vi "Playback Controls.vi"() -> ()   [LabVIEW 2020]
uses:
  <vilib>/Rock Robotics/WPI/Dashboard/WPI_DashboardPlay Operation.ctl
  <vilib>/Rock Robotics/WPI/Dashboard/WPI_DashboardLogging Global.vi
  <vilib>/Utility/inputDevices.llb/mouseAcquire.vi
panel:
  in  "Operation":u16(ring) items=["", "Rename", "Delete", "Show Folder"]
  in  "Rename":string
  in  "Dragging?":bool
  in  "Scrollbar":dbl(slide) scale=0.0..12.36
  in  "Speed":u16(ring)=3 items=["1/10 x", "1/5 x", "1/2 x", "1 x", "2 x", "5 x", "10 x"]
  in  "Playback Button":bool
  in  "Pause Button":bool
  in  "File Selector":u16(ring) items=["Select a Log File", "2017_11_07 07-17-37 Tue -- 3.2 secs", "2017_11_07 08-09-29 Tue -- 8.7 secs", "2017_11_07 08-19-10 Tue -- 11.1 secs", "2017_11_07 08-21-00 Tue -- 12.4 secs", "Test -- 2.6 secs"]
  in  "Drag Button":bool
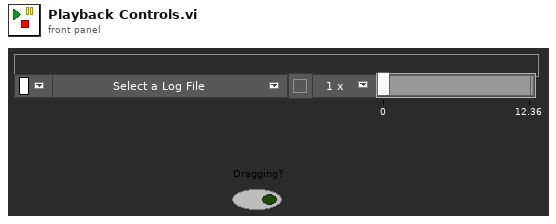
[diagram p1: front panel]
types:
  T1 = cluster{"Video 1":i32, "Video 2":i32, "Video 3":i32, "Video 4":i32}
  T2 = typedef "WPI_DashboardPlay Operation.ctl" = enum16{"Play", "Pause", "Finished"}
  T3 = typedef "LVRectTypeDef.ctl" = cluster{"Left":i16, "Top":i16, "Right":i16, "Bottom":i16}
  T4 = cluster{"Horizontal":i32, "Vertical":i32, "Scrolling":i32}
  T5 = cluster{"Horizontal":i32, "Vertical":i32, "Horizontal":i32, "Vertical":i32}
  T6 = cluster{"button 1":bool, "button 2":bool, "button 3":bool, "button 4":bool}
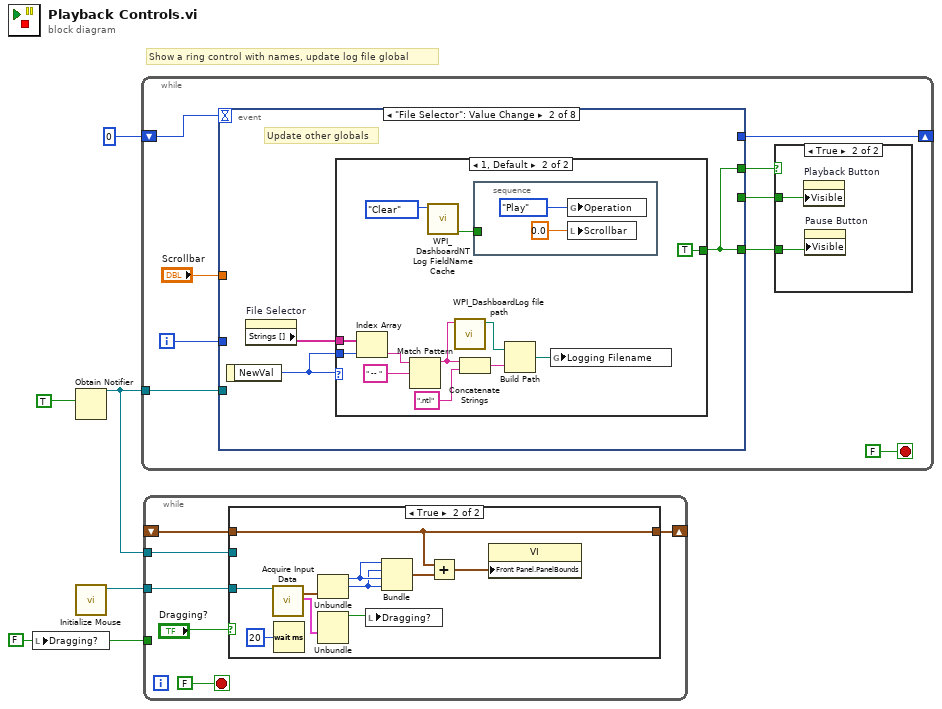
[diagram p0: block diagram]
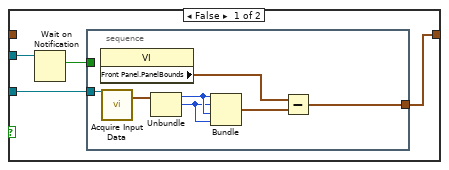
[diagram p2: hidden frame]
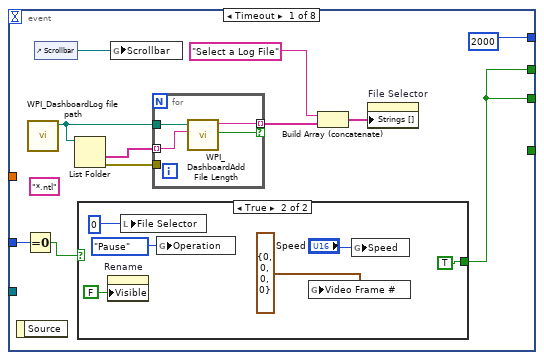
[diagram p4: hidden frame]
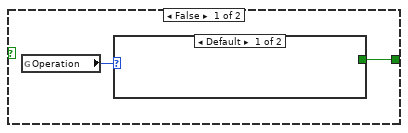
[diagram p5: hidden frame]
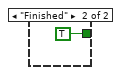
[diagram p6: hidden frame]
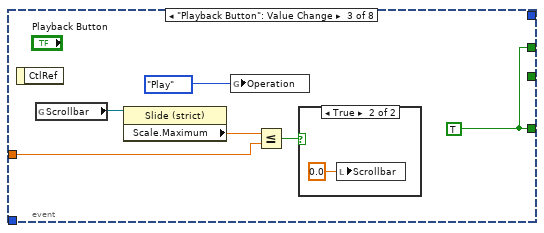
[diagram p8: hidden frame]
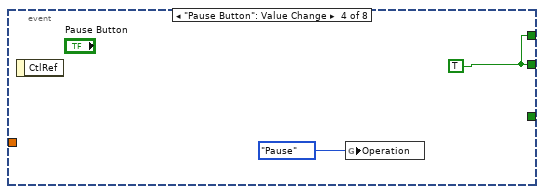
[diagram p10: hidden frame]
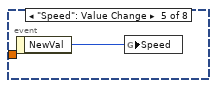
[diagram p11: hidden frame]
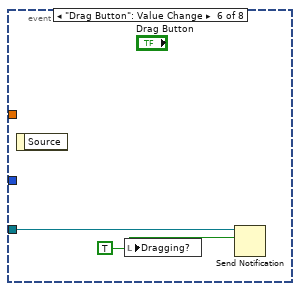
[diagram p12: hidden frame]
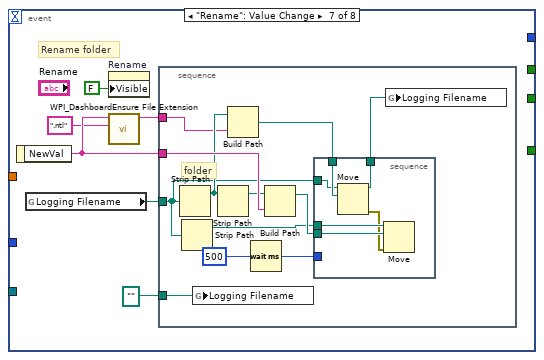
[diagram p13: hidden frame]
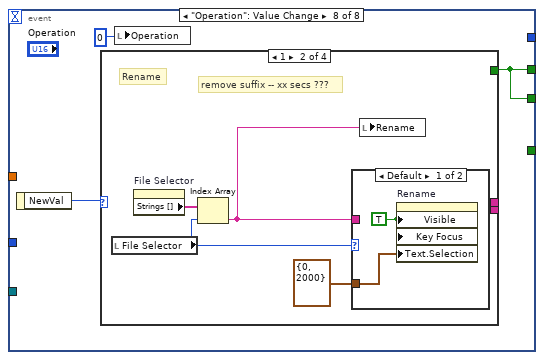
[diagram p14: hidden frame]
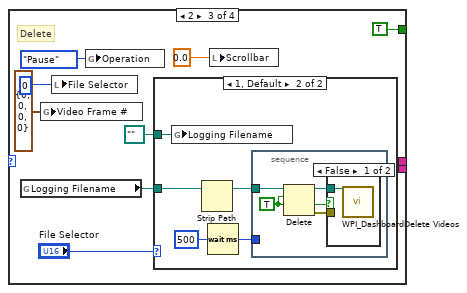
[diagram p17: hidden frame]
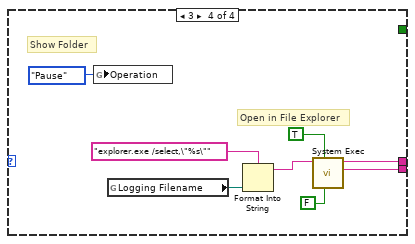
[diagram p20: hidden frame]
diagram:
  w2 = FALSE ("Dragging?")
  # "Show a ring control with names, update log file global"
  n1 = local write "Dragging?"(w2) -> ()
  n2 = Obtain Notifier(notification data type=TRUE ("Dragging?")) -> (notifier out=w3:refnum<notifier>)  [unwired: 3 in, 2 out]
  n3 = call <vilib>:"Initialize Mouse.vi"() -> ("device ID"=w4:refnum<k1>)  [unwired: 10 in, 1 out]
  n4 = while {
    shift-right: [w13] -> _
    shift-left: 0 -> [w12]
    tunnel: w3 -> [w6]
    i -> [w8]
    stop <- FALSE stop-if-true
    n5 = event shown="[1] \"File Selector\": Value Change" {
      selector: _ -> [_ _ _ _ _ _ _ _]
      dyn-events: _ -> [_ _ _ _ _ _ _ _]
      timeout: w12 -> [_ _ _ _ _ _ _ _]
      tunnel: [2000 _ _ _ _ _ _ _] -> w13
      tunnel: [_ w41 w63 _ _ _ _ _] -> w11
      tunnel: [w20 _ _ w66 _ _ _ w95] -> w10
      tunnel: [w20 w41 w63 w66 _ _ _ w95] -> w9
      tunnel: w8 -> [w22 _ _ _ _ _ _ _]
      tunnel: "Scrollbar" -> [_ _ w59 _ _ _ _ _]
      tunnel: w6 -> [_ _ _ _ _ w69 _ _]
      event Timeout {
        (unwired) "*.ntl" ("pattern")
        n6 = event-data() -> ()  [unwired: 1 in, 1 out]
        n7 = Equal To 0?(x=w22) -> (x = 0?=w21:bool)
        n8 = call <vilib>:"WPI_DashboardLog file path.vi"() -> ("appended path"=w19:path)  [unwired: 11 in]
        n9 = control-ref of="Scrollbar"() -> (w26:refnum<vi>)
        n10 = List Folder(path=w19) -> (folder names=w17:string[], error out=w18:errorcluster)  [unwired: 3 in, 2 out]
        n11 = case shown="True" w21 {
          tunnel: [w28 TRUE] -> w20
          frame False {
            n12 = global read "WPI_DashboardLogging Global.vi" "Operation"() -> (w29:T2)
            n13 = case shown="Default" w29 {
              tunnel: [_ TRUE] -> w28
              frame Default {
              }
              frame "Finished" {
              }
            }
          }
          frame True {
            n14 = property on="Rename" class="Str"("Visible"=FALSE) -> ()  [unwired: 2 in, 2 out]
            n15 = local write "File Selector"(0) -> ()
            n16 = global write "WPI_DashboardLogging Global.vi" "Operation"(WPI_DashboardPlay_Operation."Pause" ("Operation")) -> ()
            n17 = global write "WPI_DashboardLogging Global.vi" "Video Frame #"(T1 {"Video 1"=0, "Video 2"=0, "Video 3"=0, "Video 4"=0} ("Video Frame #")) -> ()
            n18 = global write "WPI_DashboardLogging Global.vi" "Speed"("Speed") -> ()
          }
        }
        n19 = global write "WPI_DashboardLogging Global.vi" "Scrollbar"(w26) -> ()
        n20 = for {
          tunnel: w17 -> [w38] mode=indexing
          tunnel: [w40] -> w25 mode=indexing if=w37
          tunnel: w19 -> [w39]
          tunnel: w18 -> [_]
          n21 = call <vilib>:"WPI_DashboardAdd File Length.vi"("String in"=w38, "appended path"=w39) -> ("Valid"=w37:bool, "String out"=w40:string)  [unwired: 8 in]
        }
        n22 = Build Array (concatenate)("Select a Log File" ("pattern"), w25) -> (w24:string[])
        n23 = property on="File Selector" class="Ring (strict)"("Strings []"=w24) -> ()  [unwired: 2 in, 2 out]
      }
      event "File Selector": Value Change {
        # "Update other globals"
        n24 = event-data() -> ("NewVal"=w42:u16)  [unwired: 1 in]
        n25 = property on="File Selector" class="Ring (strict)"() -> ("Strings []"=w43:string[])  [unwired: 2 in, 2 out]
        n26 = case shown="1, Default" w42 {
          tunnel: w43 -> [_ w55]
          tunnel: w42 -> [_ w54]
          tunnel: [_ TRUE ("Visible")] -> w41
          frame 0 {
          }
          frame 1, Default {
            n27 = Index Array(array=w55, index=w54) -> (element=w49:string)
            n28 = Match Pattern(string=w49, regular expression=" -- ") -> (before substring=w44:string)  [unwired: 1 in, 3 out]
            n29 = call <vilib>:"WPI_DashboardNT Log FieldName Cache.vi"("Operation"=enum16{"Lookup/Add", "Index", "Clear"}."Clear") -> ("New/Valid"=w46:bool)  [unwired: 8 in, 2 out]
            n30 = call <vilib>:"WPI_DashboardLog file path.vi"("Time Date String"=w44) -> ("appended path"=w53:path)  [unwired: 10 in]
            n31 = Concatenate Strings(w44, ".ntl") -> (w51:string)
            n32 = stacked-sequence {
              tunnel: w46 -> [_]
              frame #0 {
                n33 = global write "WPI_DashboardLogging Global.vi" "Operation"(WPI_DashboardPlay_Operation."Play" ("Operation")) -> ()
                n34 = local write "Scrollbar"(0.0 ("Position")) -> ()
              }
            }
            n35 = Build Path(base path=w53, name or relative path=w51) -> (appended path=w50:path)
            n36 = global write "WPI_DashboardLogging Global.vi" "Logging Filename"(w50) -> ()
          }
        }
      }
      event "Playback Button": Value Change {
        w63 = TRUE ("Visible")
        n37 = event-data() -> ()  [unwired: 1 in, 1 out]
        n38 = global read "WPI_DashboardLogging Global.vi" "Scrollbar"() -> (w61:refnum<vi>)
        n39 = property class="Slide (strict)"(reference=w61) -> ("Scale.Maximum"=w60:dbl)  [unwired: 1 in, 2 out]
        n40 = global write "WPI_DashboardLogging Global.vi" "Operation"(WPI_DashboardPlay_Operation."Play" ("Operation")) -> ()
        n41 = Less Or Equal?(x=w60, y=w59) -> (x <= y?=w58:bool)
        n42 = case shown="True" w58 {
          frame False {
          }
          frame True {
            n43 = local write "Scrollbar"(0.0 ("Scrollbar")) -> ()
          }
        }
      }
      event "Pause Button": Value Change {
        w66 = TRUE ("Visible")
        n44 = event-data() -> ()  [unwired: 1 in, 1 out]
        n45 = global write "WPI_DashboardLogging Global.vi" "Operation"(WPI_DashboardPlay_Operation."Pause" ("Operation")) -> ()
      }
      event "Speed": Value Change {
        n46 = event-data() -> ("NewVal"=w67:u16)  [unwired: 1 in]
        n47 = global write "WPI_DashboardLogging Global.vi" "Speed"(w67) -> ()
      }
      event "Drag Button": Value Change {
        w68 = TRUE ("Dragging?")
        n48 = event-data() -> ()  [unwired: 1 in, 1 out]
        n49 = local write "Dragging?"(w68) -> ()
        n50 = Send Notification(notification=w68, notifier=w69) -> ()  [unwired: 1 in, 2 out]
      }
      event "Rename": Value Change {
        # "Rename folder"
        n51 = event-data() -> ("NewVal"=w72:string)  [unwired: 1 in]
        n52 = global read "WPI_DashboardLogging Global.vi" "Logging Filename"() -> (w74:path)
        n53 = property on="Rename" class="Str"("Visible"=FALSE) -> ()  [unwired: 2 in, 2 out]
        n54 = call <vilib>:"WPI_DashboardEnsure File Extension.vi"("Extension"=".ntl", "Name"=w72) -> ("Name Out"=w70:string)  [unwired: 9 in]
        n55 = stacked-sequence {
          tunnel: w72 -> [w83]
          tunnel: w74 -> [w76]
          tunnel: path "" ("Logging Filename") -> [w86]
          tunnel: w70 -> [w78]
          frame #0 {
            # "folder"
            n56 = Strip Path(path=w76) -> (stripped path=w79:path)  [unwired: 1 out]
            n57 = Strip Path(path=w76) -> (stripped path=w80:path)  [unwired: 1 out]
            n58 = global write "WPI_DashboardLogging Global.vi" "Logging Filename"(w86) -> ()
            n59 = Strip Path(path=w79) -> (stripped path=w81:path)  [unwired: 1 out]
            n60 = Build Path(base path=w79, name or relative path=w78) -> (appended path=w77:path)
            n61 = Wait (ms)(milliseconds to wait=u32 500) -> (millisecond timer value=w84:u32)
            n62 = Build Path(base path=w81, name or relative path=w83) -> (appended path=w87:path)
            n63 = stacked-sequence {
              tunnel: w87 -> [w93]
              tunnel: w80 -> [w92]
              tunnel: w84 -> [_]
              tunnel: [w90] -> w82
              tunnel: w77 -> [w91]
              tunnel: w76 -> [w89]
              frame #0 {
                n64 = Move(source path=w89, 10:w91) -> (error out=w88:errorcluster, 3:w90:path)  [unwired: 3 in, 1 out]
                n65 = Move(source path=w92, error in=w88, 10:w93) -> ()  [unwired: 2 in, 3 out]
              }
            }
            n66 = global write "WPI_DashboardLogging Global.vi" "Logging Filename"(w82) -> ()
          }
        }
      }
      event "Operation": Value Change {
        n67 = event-data() -> ("NewVal"=w96:u16)  [unwired: 1 in]
        n68 = case shown="1" w96 {
          tunnel: [_ _ TRUE _] -> w95
          tunnel: [_ _ _ w125] -> _
          tunnel: [_ _ _ w124] -> _
          frame 0, Default {
          }
          frame 1 {
            # "remove suffix -- xx secs ???"
            # "Rename"
            n69 = local read "File Selector"() -> (w98:u16)
            n70 = property on="File Selector" class="Ring (strict)"() -> ("Strings []"=w100:string[])  [unwired: 2 in, 2 out]
            n71 = Index Array(array=w100, index=w98) -> (element=w99:string)
            n72 = case shown="Default" w98 {
              tunnel: w99 -> [_ _]
              tunnel: cluster{i32, i32} {0, 2000} -> [w101 _]
              frame Default {
                w102 = TRUE ("Visible")
                n73 = property on="Rename" class="Str"("Visible"=w102, "Key Focus"=w102, "Text.Selection"=w101) -> ()  [unwired: 2 in, 2 out]
              }
              frame 0 {
              }
            }
            n74 = local write "Rename"(w99) -> ()
          }
          frame 2 {
            # "Delete"
            n75 = global read "WPI_DashboardLogging Global.vi" "Logging Filename"() -> (w106:path)
            n76 = global write "WPI_DashboardLogging Global.vi" "Video Frame #"(T1 {"Video 1"=0, "Video 2"=0, "Video 3"=0, "Video 4"=0} ("Video Frame #")) -> ()
            n77 = local write "File Selector"(0) -> ()
            n78 = global write "WPI_DashboardLogging Global.vi" "Operation"(WPI_DashboardPlay_Operation."Pause" ("Operation")) -> ()
            n79 = case shown="1, Default" "File Selector" {
              tunnel: w106 -> [_ w112]
              tunnel: path "" ("Logging Filename") -> [_ w115]
              frame 0 {
              }
              frame 1, Default {
                n80 = global write "WPI_DashboardLogging Global.vi" "Logging Filename"(w115) -> ()
                n81 = Strip Path(path=w112) -> (stripped path=w111:path)  [unwired: 1 out]
                n82 = Wait (ms)(milliseconds to wait=u32 500) -> (millisecond timer value=w113:u32)
                n83 = stacked-sequence {
                  tunnel: w111 -> [w120]
                  tunnel: w113 -> [_]
                  frame #0 {
                    w117 = TRUE ("confirm (F)")
                    n84 = Delete(path (use dialog)=w120, entire hierarchy (F)=w117, confirm (F)=w117) -> (deleted path=w118:path, cancelled=w119:bool, error out=w116:errorcluster)  [unwired: 2 in]
                    n85 = case shown="False" w119 {
                      tunnel: w118 -> [w121 _]
                      tunnel: w116 -> [_ _]
                      frame False {
                        n86 = call <vilib>:"WPI_DashboardDelete Videos.vi"("Path"=w121) -> ()  [unwired: 11 in]
                      }
                      frame True {
                      }
                    }
                  }
                }
              }
            }
            n87 = local write "Scrollbar"(0.0 ("Position")) -> ()
          }
          frame 3 {
            # "Open in File Explorer"
            # "Show Folder"
            n88 = global write "WPI_DashboardLogging Global.vi" "Operation"(WPI_DashboardPlay_Operation."Pause" ("Operation")) -> ()
            n89 = global read "WPI_DashboardLogging Global.vi" "Logging Filename"() -> (w122:path)
            n90 = Format Into String(format string="explorer.exe /select,\"%s\"", w122) -> (resulting string=w128:string)  [unwired: 2 in, 1 out]
            n91 = call <vilib>:"System Exec.vi"("run minimized? (F)"=FALSE, "wait until completion? (T)"=TRUE, "command line"=w128) -> ("standard error"=w125:string, "standard output"=w124:string)  [unwired: 5 in, 2 out]
          }
        }
        n92 = local write "Operation"(0) -> ()
      }
    }
    n93 = case shown="True" w9 {
      tunnel: w11 -> [_ w16]
      tunnel: w10 -> [_ w15]
      frame False {
      }
      frame True {
        n94 = property on="Playback Button" class="Bool"("Visible"=w15) -> ()  [unwired: 2 in, 2 out]
        n95 = property on="Pause Button" class="Bool"("Visible"=w16) -> ()  [unwired: 2 in, 2 out]
      }
    }
  }
  n96 = while {
    tunnel: w4 -> [w135]
    tunnel: w3 -> [w133]
    tunnel: w2 -> [_]
    shift-right: [w131] -> _
    shift-left: _ -> [w130]
    stop <- FALSE stop-if-true
    n97 = case shown="True" "Dragging?" {
      tunnel: w135 -> [w138 w156]
      tunnel: w133 -> [w139 _]
      tunnel: [w137 w148] -> w131
      tunnel: w130 -> [_ w148]
      frame False {
        n98 = Wait on Notification(notifier=w139) -> (notification=w136:bool)  [unwired: 3 in, 3 out]
        n99 = stacked-sequence {
          tunnel: w138 -> [w146]
          tunnel: [w142] -> w137
          tunnel: w136 -> [_]
          frame #0 {
            n100 = property class="VI"() -> ("Front Panel.PanelBounds"=w144:T3)  [unwired: 2 in, 2 out]
            n101 = call-poly <vilib>:"Acquire Input Data.vi"("device ID"=w146) -> ("axis info"=w145:T4)  [unwired: 15 in, 3 out]
            n102 = Unbundle(w145) -> ("Horizontal"=w141:i32, "Vertical"=w140:i32)  [unwired: 1 out]
            n103 = Bundle("Horizontal"=w141, "Vertical"=w140, "Horizontal"=w141, "Vertical"=w140) -> (w143:T5)  [unwired: 1 in]
            n104 = Subtract(x=w144, y=w143) -> (x-y=w142:cluster{i32, i32, i32, i32})
          }
        }
      }
      frame True {
        n105 = call-poly <vilib>:"Acquire Input Data.vi"("device ID"=w156) -> ("axis info"=w152:T4, "button info"=w154:T6)  [unwired: 15 in, 2 out]
        n106 = Wait (ms)(milliseconds to wait=u32 20) -> ()  [unwired: 1 out]
        n107 = Unbundle(w152) -> ("Horizontal"=w151:i32, "Vertical"=w150:i32)  [unwired: 1 out]
        n108 = Unbundle(w154) -> ("button 1"=w153:bool)  [unwired: 3 out]
        n109 = local write "Dragging?"(w153) -> ()
        n110 = Bundle("Horizontal"=w151, "Vertical"=w150, "Horizontal"=w151, "Vertical"=w150) -> (w149:T5)  [unwired: 1 in]
        n111 = Add(x=w148, y=w149) -> (x+y=w147:cluster{i32, i32, i32, i32})
        n112 = property class="VI"("Front Panel.PanelBounds"=w147) -> ()  [unwired: 2 in, 2 out]
      }
    }
  }
